vi "DSF.Engine.Execution.Builder.Run.vi"(8 "error in (no error)":errorcluster, 11 "Builder in":refnum<class "DSF.Engine.Execution.Builder.lvclass">) -> (0 "error out":errorcluster, 3 "Builder out":refnum<class "DSF.Engine.Execution.Builder.lvclass">)   [LabVIEW 2016, in "DSF.Engine.lvlib" / "DSF.Engine.Execution.Builder.lvclass"]
uses:
  DSF.Engine.Execution.Builder.lvclass
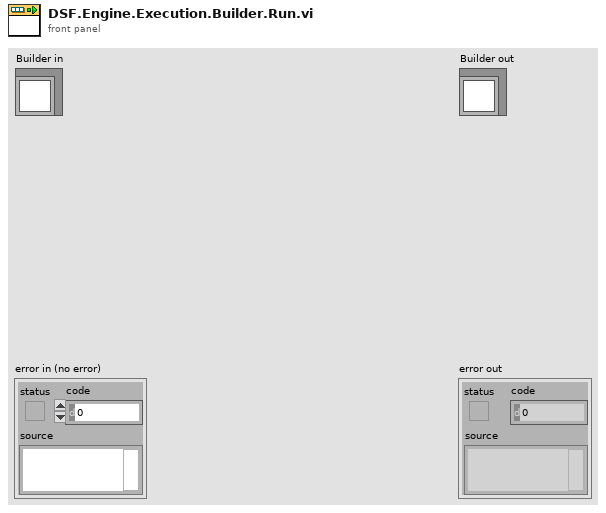
[diagram p1: front panel]
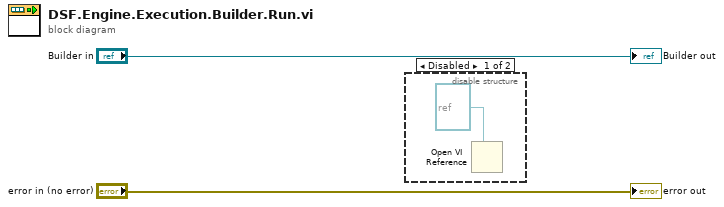
[diagram p0: block diagram]
diagram:
  n1 = disable-structure shown="Disabled" {
    frame Disabled {
      n2 = Open VI Reference(type specifier VI Refnum (for type only)=refnum<vi> refnum) -> ()  [unwired: 5 in, 2 out]
    }
    frame Enabled {
    }
  }
  "error out" <- "error in (no error)"
  "Builder out" <- "Builder in"
